vi "Send Target Command.vi"(7 "Instrument":string, 8 "error in":errorcluster, 9 "Value":variant, 10 "Command":string, 11 "Launcher in":refnum<class "Launcher.lvclass">) -> (0 "error out":errorcluster, 3 "Launcher out":refnum<class "Launcher.lvclass">)   [LabVIEW 2019, in "Launcher.lvlib" / "Launcher.lvclass"]
uses:
  Library/Launcher.lvclass
  builds/Instruments/Instruments.lvlibp/Instruments Messages/Send Command Msg/Send Command Msg.lvclass
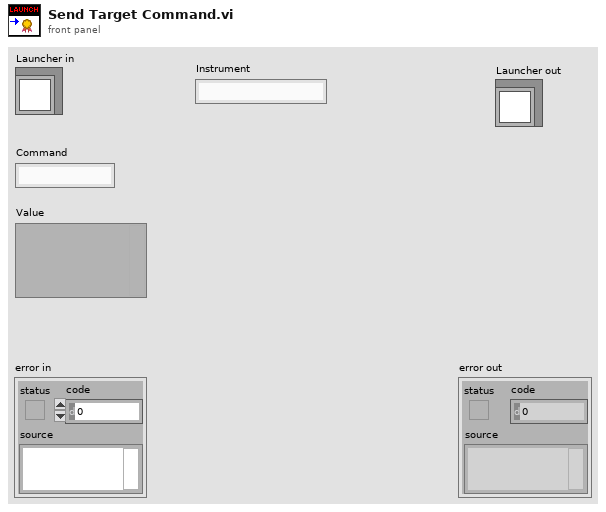
[diagram p1: front panel]
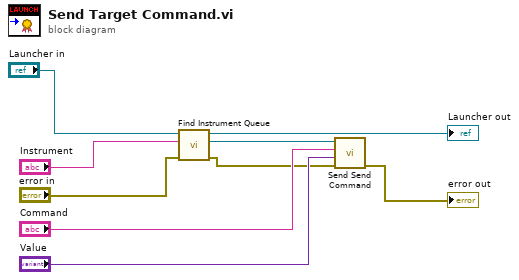
[diagram p0: block diagram]
diagram:
  n1 = call "Find Instrument Queue.vi"("error in"="error in", "Instrument"="Instrument", "Launcher in"="Launcher in") -> ("error out"=w1:errorcluster, "Queue"=w4:refnum<class "Message Enqueuer.lvclass">, "Launcher out"=→"Launcher out":refnum<class "Launcher.lvclass">)  [unwired: 6 in]
  n2 = call "Send Send Command.vi"("error in (no error)"=w1, "Value"="Value", "Command"="Command", "Message Enqueuer"=w4) -> ("error out"=→"error out":errorcluster)  [unwired: 6 in, 1 out]
